vi "Read database.vi"(5 "String":string) -> (0 "error out":errorcluster, 1 "Operator Code":string[](array[string]), 2 "DB Data":T1)   [LabVIEW 2020]
uses:
  <vilib>/addons/database/Connection.llb/DB Tools Open Connec (String).vi
  Galobal variable_TI.vi
  <vilib>/addons/database/_DB Variant To Data/Database Variant To Data.xnode
  <vilib>/addons/database/NI_Database_API.lvlib
panel:
  out "data":string[][](array[string])
  out "appended array 4":string[](array[string])
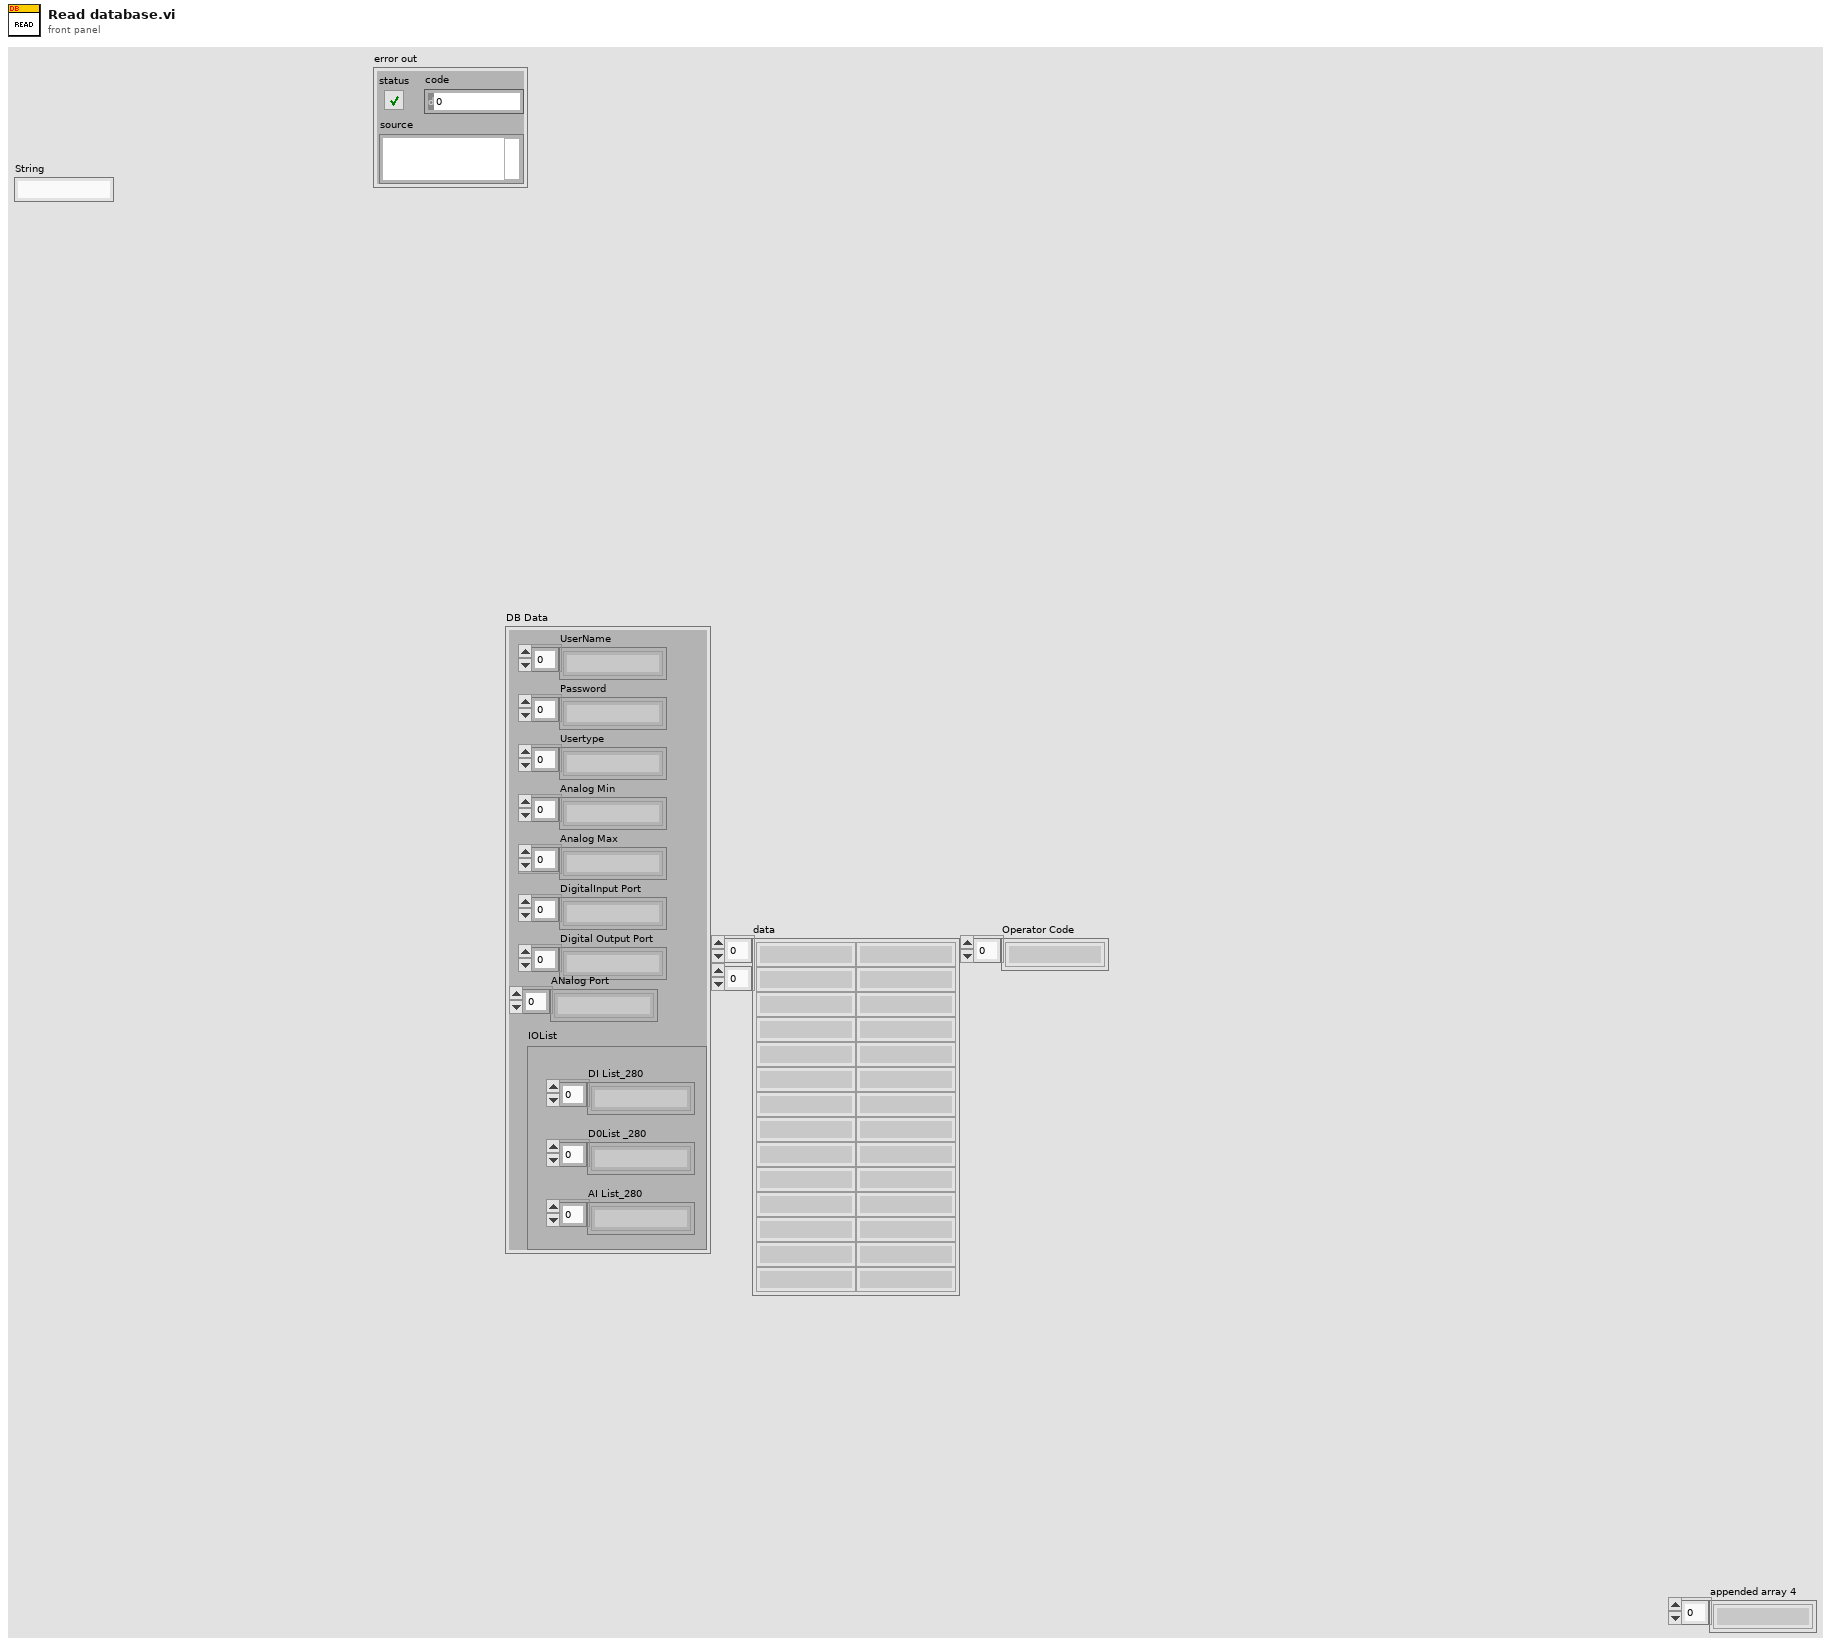
[diagram p1: front panel]
types:
  T1 = cluster{"UserName":string[], "Password":string[], "Usertype":string[], "Analog Min":string[], "Analog Max":string[], "DigitalInput Port":string[], "Digital Output Port":string[], "ANalog Port":string[], "IOList":cluster{"DI List_280":string[], "D0List _280":string[], "AI List_280":string[]}}
  T2 = cluster{"ILSensormax_1":dbl, "ILSensormin_1":dbl, "ILSensormax _2":dbl, "ILSensormin_2":dbl}
  T3 = cluster{"To-A":timestamp, "From-A":timestamp, "From-B":timestamp, "To-B":timestamp, "From-C 1":timestamp, "To-C 1":timestamp, "From-C 2":timestamp, "To-C 2":timestamp, "Shift":string}[]
  T4 = typedef "NI_Database_API.lvlib/Conn ObjectReference.ctl" = refnum<k1>
  T5 = cluster{"DI List_280":string[], "D0List _280":string[], "AI List_280":string[]}
  T6 = cluster{"To-A":timestamp, "From-A":timestamp, "From-B":timestamp, "To-B":timestamp, "From-C 1":timestamp, "To-C 1":timestamp, "From-C 2":timestamp, "To-C 2":timestamp, "Shift":string}
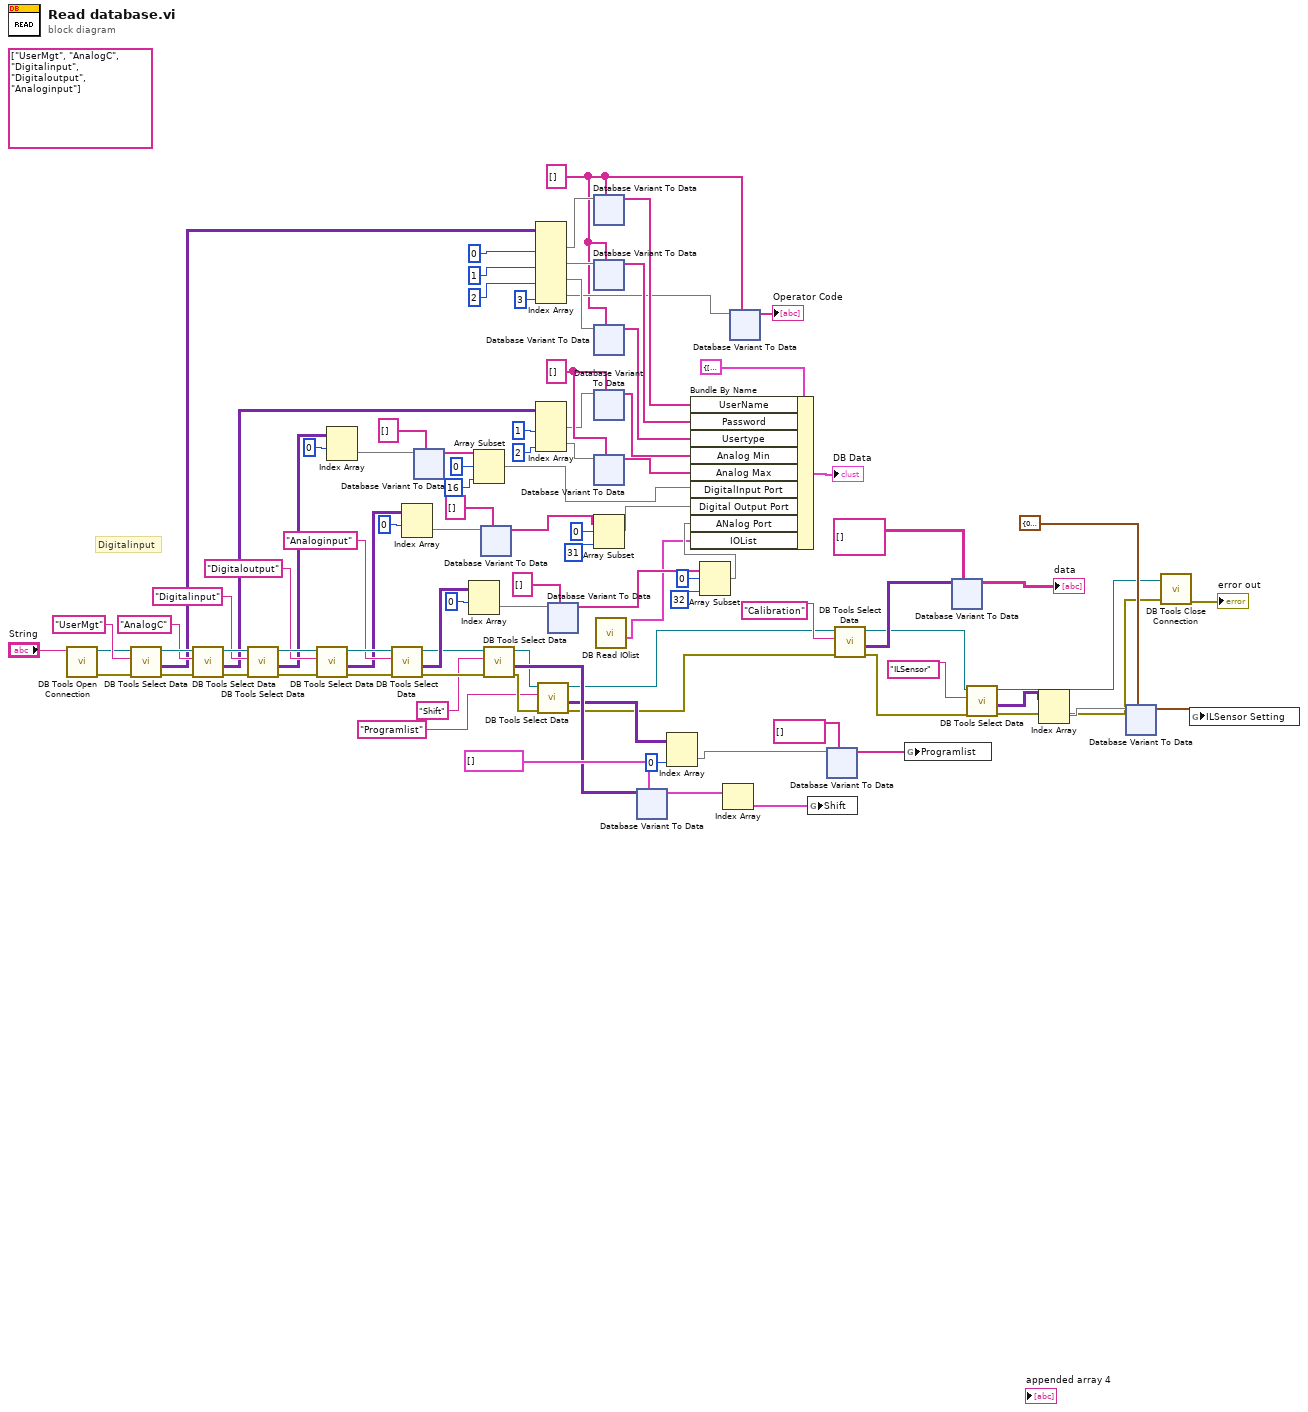
[diagram p0: block diagram]
diagram:
  w87 = string[] []
  (unwired) string[] ["UserMgt", "AnalogC", "Digitalinput", "Digitaloutput", "Analoginput"]
  w2 = string[] []
  # "Digitalinput"
  n1 = call-poly <vilib>:"DB Tools Open Connection.vi"("connection information"="String") -> ("error out"=w55:errorcluster, "connection reference"=w56:T4)  [unwired: 7 in]
  n2 = call <vilib>:"DB Tools Select Data.vi"("error in (no error)"=w55, "table"="UserMgt", "connection reference"=w56) -> ("error out"=w69:errorcluster, "data"=w54:variant[][], "connection reference out"=w67:T4)  [unwired: 3 in]
  n3 = call <vilib>:"DB Tools Select Data.vi"("error in (no error)"=w69, "table"="AnalogC", "connection reference"=w67) -> ("error out"=w68:errorcluster, "data"=w53:variant[][], "connection reference out"=w66:T4)  [unwired: 3 in]
  n4 = call <vilib>:"DB Tools Select Data.vi"("error in (no error)"=w68, "table"="Digitalinput", "connection reference"=w66) -> ("error out"=w62:errorcluster, "data"=w52:variant[][], "connection reference out"=w61:T4)  [unwired: 3 in]
  n5 = call <vilib>:"DB Tools Select Data.vi"("error in (no error)"=w62, "table"="Digitaloutput", "connection reference"=w61) -> ("error out"=w58:errorcluster, "data"=w51:variant[][], "connection reference out"=w59:T4)  [unwired: 3 in]
  n6 = Index Array(array=w52, index (row)=0 ("disabled index (col)")) -> (element=w89:variant[])  [unwired: 1 in]
  n7 = call <vilib>:"DB Tools Select Data.vi"("error in (no error)"=w58, "table"="Analoginput", "connection reference"=w59) -> ("error out"=w45:errorcluster, "data"=w50:variant[][], "connection reference out"=w44:T4)  [unwired: 3 in]
  n8 = Index Array(array=w51, index (row)=0 ("disabled index (col)")) -> (element=w90:variant[])  [unwired: 1 in]
  n9 = xnode "Database Variant To Data"("database variant"=w89, "type"=string[] []) -> ("data"=w41:string[])  [unwired: 1 in, 1 out]
  n10 = Index Array(array=w50, index (row)=0 ("disabled index (col)")) -> (element=w93:variant[])  [unwired: 1 in]
  n11 = Array Subset(array=w41, index=0, length=16) -> (w38:string[])
  n12 = xnode "Database Variant To Data"("database variant"=w90, "type"=string[] []) -> ("data"=w36:string[])  [unwired: 1 in, 1 out]
  n13 = call <vilib>:"DB Tools Select Data.vi"("error in (no error)"=w45, "table"="Shift", "connection reference"=w44) -> ("error out"=w27:errorcluster, "data"=w42:variant[][], "connection reference out"=w28:T4)  [unwired: 3 in]
  n14 = Index Array(array=w54, index (col) #1=0 ("disabled index (col)"), index (col) #2=1 ("index (col)"), index (col) #3=2 ("index (col)"), index (col) #4=3 ("index (col)")) -> (element #1=w80:variant[], element #2=w77:variant[], element #3=w76:variant[], element #4=w3:variant[])  [unwired: 4 in]
  n15 = Index Array(array=w53, index (col) #1=1 ("disabled index (col)"), index (col) #2=2 ("index (col)")) -> (element #1=w85:variant[], element #2=w86:variant[])  [unwired: 2 in]
  n16 = call <vilib>:"DB Tools Select Data.vi"("error in (no error)"=w27, "table"="Programlist", "connection reference"=w28) -> ("error out"=w18:errorcluster, "data"=w25:variant[][], "connection reference out"=w19:T4)  [unwired: 3 in]
  n17 = xnode "Database Variant To Data"("database variant"=w93, "type"=string[] []) -> ("data"=w31:string[])  [unwired: 1 in, 1 out]
  n18 = xnode "Database Variant To Data"("database variant"=w80, "type"=w2) -> ("data"=w75:string[])  [unwired: 1 in, 1 out]
  n19 = xnode "Database Variant To Data"("database variant"=w77, "type"=w2) -> ("data"=w74:string[])  [unwired: 1 in, 1 out]
  n20 = xnode "Database Variant To Data"("database variant"=w76, "type"=w2) -> ("data"=w73:string[])  [unwired: 1 in, 1 out]
  n21 = xnode "Database Variant To Data"("database variant"=w85, "type"=w87) -> ("data"=w72:string[])  [unwired: 1 in, 1 out]
  n22 = xnode "Database Variant To Data"("database variant"=w86, "type"=w87) -> ("data"=w71:string[])  [unwired: 1 in, 1 out]
  n23 = Array Subset(array=w36, index=0, length=31) -> (w34:string[])
  n24 = call "DB Read IOlist.vi"() -> ("output cluster"=w29:T5)  [unwired: 11 in]
  n25 = xnode "Database Variant To Data"("database variant"=w42, "type"=T3 []) -> ("data"=w46:T3)  [unwired: 1 in, 1 out]
  n26 = Index Array(array=w25, index (col)=0 ("disabled index (col)")) -> (element=w24:variant[])  [unwired: 1 in]
  n27 = Array Subset(array=w31, index=0, length=32) -> (w30:string[])
  n28 = Bundle By Name(cluster=T1 {"UserName"=[], "Password"=[], "Usertype"=[], "Analog Min"=[], "Analog Max"=[], "DigitalInput Port"=[], "Digital Output Port"=[], "ANalog Port"=[], "IOList"={"DI List_280"=[" Start PB (P0.0) ", "Emergency Stop (P0.1)", "Reset PB (P0.2)", "Home PB (P0.3)", "Main Pressure Signal (P0.4)", "Safety Signal-1 (P0.5)", "Safety Signal-2 (P0.6)", "Fixture Sliding Servo Home RS (P0.7)", "Fixture Sliding Servo Fault Signal (P0.8)", "LCD pressing Servo Home RS (P0.9)", "LCD pressing Servo fault Signal (P0.10)", "Spare", "Spare", "Spare", "Spare", "Model conformation PX-1 (AI2)", "Model conformation PX-2 (AI3)", "Diffuser height checking Sensor-1 (AI4)", "Diffuser height checking Sensor-2 (AI5)", "Panel Door Open Signal (AI6)", "Component CNF Sensor on Ionizer (AI7)", "Bi-adhesive tube Waste Collection bin CNF Sensor (AI8)", "Photo Prism presence Sensor (AI9)", "Lightbox presence CNF Sensor (AI10)", "Diffuser presence CNF Sensor (AI11)", "Photo prism height checking UP CYL Rs (AI12)", "Photo prism height checking DWN CYL  Rs (AI13)", "Camera slide Cyl Fwd Rs (AI14)", "Camera slide Cyl Rev Rs (AI15)", "LCD Display Rotating Unit Actuator Cyl CW PX (AI16)", "LCD Display Rotating Unit Actuator Cyl CCW PX (AI17)", "Fixture clamping Cyl Fwd Rs (AI18)", "Fixture clamping Cyl Rev Rs (AI19)", "Clip pulling unit Cyl Fwd Rs (AI20)", "Clip pulling unit Cyl Rev Rs (AI21)", "Clip clamp unit Cyl Fwd Rs (A22)", "Clip clamp unit Cyl Rev Rs (AI23)", "Barcode Scanner Ready Signal (AI24)", "Spare", "Spare", "Spare", "Spare", "Spare", "Spare", "Spare"], "D0List _280"=["Ionizer ON Sol (P0.16)", "Fixture Slide Servo Fault Reset (P0.17)", "LCD pressing servo Fault Reset (P0.18)", "Fixture Slide servo Brake ON Cmd (P0.19)", "Fixture Slide Servo Direction Command (P0.20)", "LCD pressing Servo Direction Command (P0.21)", "LCD pressing Servo Brake ON Cmd (P0.22)", "Photo prism height checking UP CYL Sol (P0.23)", "Photo prism height checking DWN CYL  Sol (P0.24)", "Camera slide Cyl Fwd Sol (P0.25)", "Camera slide Cyl Rev Sol (P0.26)", "LCD Display Rotating Unit Actuator Cyl CW Sol (P0.27)", "LCD Display Rotating Unit Actuator Cyl CCW Sol (P0.28)", "Fixture clamping Cyl Fwd Sol (P0.29)", "Fixture clamping Cyl Rev Sol (P0.30)", "Clip pulling unit Cyl Fwd Sol (P0.31)", "Clip pulling unit Cyl Rev Sol (P1.0)", "Clip clamp unit Cyl Up Sol (P1.1)", "Clip clamp unit Cyl Dwn Sol (P1.2)", "Optional required based Barcode Trigger Cmd (P1.3)", "TWL Red /Fault with Buzzer (P1.4)", "TWL Green/OK (P1.5)", "TWL Yellow/ Running (P1.6)", "Spare", "Spare", "Spare", "Spare", "Spare", "Fixture Slide Servo Pulse Command (P2.4)", "LCD pressing Servo Pulse Command (P2.5)", "Spare", "Spare"], "AI List_280"=["Loadcell Signal For LCD PRESSING (AI0)", "LVDT SIGNAL FOR PHOTO PRISM HEIGHT CHECK (AI1)"]}} ("DB Data 2"), "UserName"=w75, "Password"=w74, "Usertype"=w73, "Analog Min"=w72, "Analog Max"=w71, "DigitalInput Port"=w38, "Digital Output Port"=w34, "ANalog Port"=w30, "IOList"=w29) -> (→"DB Data":T1)
  n29 = Index Array(array=w46) -> (element=w5:T6)  [unwired: 1 in]
  n30 = xnode "Database Variant To Data"("database variant"=w3, "type"=w2) -> ("data"=→"Operator Code":string[])  [unwired: 1 in, 1 out]
  n31 = global write "Galobal variable_TI.vi" "Shift"(w5) -> ()
  n32 = xnode "Database Variant To Data"("database variant"=w24, "type"=string[] []) -> ("data"=w22:string[])  [unwired: 1 in, 1 out]
  n33 = call <vilib>:"DB Tools Select Data.vi"("error in (no error)"=w18, "table"="Calibration", "connection reference"=w19) -> ("error out"=w12:errorcluster, "data"=w17:variant[][], "connection reference out"=w13:T4)  [unwired: 3 in]
  n34 = global write "Galobal variable_TI.vi" "Programlist"(w22) -> ()
  n35 = xnode "Database Variant To Data"("database variant"=w17, "type"=string[][] []) -> ("data"=→"data":string[][])  [unwired: 1 in, 1 out]
  n36 = call <vilib>:"DB Tools Select Data.vi"("error in (no error)"=w12, "table"="ILSensor", "connection reference"=w13) -> ("error out"=w6:errorcluster, "data"=w11:variant[][], "connection reference out"=w7:T4)  [unwired: 3 in]
  n37 = Index Array(array=w11) -> (element=w10:variant[])  [unwired: 2 in]
  n38 = xnode "Database Variant To Data"("database variant"=w10, "type"=T2 {"ILSensormax_1"=0.0, "ILSensormin_1"=0.0, "ILSensormax _2"=0.0, "ILSensormin_2"=0.0} ("ILSensor Setting")) -> ("data"=w8:T2)  [unwired: 1 in, 1 out]
  n39 = call <vilib>:"DB Tools Close Connection.vi"("error in (no error)"=w6, "connection reference"=w7) -> ("error out"=→"error out":errorcluster)  [unwired: 5 in]
  n40 = global write "Galobal variable_TI.vi" "ILSensor Setting"(w8) -> ()
